vi "RemoveByName.vi"(8 "error in (no error)":errorcluster, 10 "Name":string, 11 "Collection in":refnum<class "CollectionByValue.lvclass">) -> (0 "error out":errorcluster, 1 "found":bool, 2 "LabVIEW Object Removed":refnum<class>, 3 "Collection out":refnum<class "CollectionByValue.lvclass">)   [LabVIEW 2021, in "Collection.lvlib" / "CollectionByValue.lvclass"]
uses:
  CollectionByValue.lvclass
  CollectionByValue.lvclass/CollectionByValue.ctl
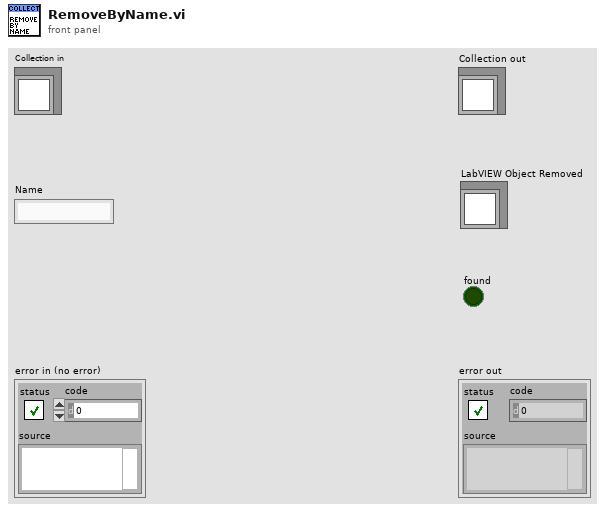
[diagram p1: front panel]
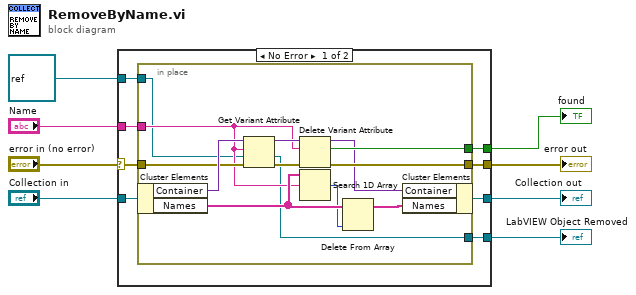
[diagram p0: block diagram]
diagram:
  n1 = case shown="No Error" "error in (no error)" {
    selector: "error in (no error)" -> [w12 w32]
    tunnel: [w11 w32] -> w7
    tunnel: [w15 w31] -> w5
    tunnel: "Collection in" -> [w16 w31]
    tunnel: "Name" -> [w14 _]
    tunnel: [w13 _] -> w3
    tunnel: refnum<class> refnum ("LabVIEW Object") -> [w10 w30]
    tunnel: [w9 w30] -> w1
    frame No Error {
      n2 = in-place {
        in-place-border: w14 -> [w19]
        in-place-border: [w26] -> w13
        in-place-border: w12 -> [w21]
        in-place-border: [w25] -> w11
        in-place-border: w10 -> [w18]
        in-place-border: [w17] -> w9
        n3 = in-place-cluster #1(w16) -> ("Container"=w23:variant, "Names"=w29:string[])
        n4 = Get Variant Attribute(Variant=w23, name=w19, default value (empty Variant)=w18, error in=w21) -> (duplicate Variant=w22:variant, value=w17:refnum<class>, error out=w20:errorcluster)  [unwired: 1 out]
        n5 = Delete Variant Attribute(4:w20, 6:w19, 7:w22) -> (0:w25:errorcluster, 2:w26:bool, 3:w24:variant)
        n6 = Search 1D Array(1D array=w29, element=w19) -> (index of element=w27:i32)  [unwired: 1 in]
        n7 = Delete From Array(array=w29, index=w27) -> (array with subset deleted=w28:string[])  [unwired: 1 in, 1 out]
        n8 = in-place-cluster #1("Container"=w24, "Names"=w28) -> (w15:refnum<class "CollectionByValue.lvclass">)
      }
    }
    frame Error {
    }
  }
  "error out" <- w7
  "Collection out" <- w5
  "found" <- w3
  "LabVIEW Object Removed" <- w1
